vi "I2C Write Byte.vi"(8 "error in (no error)":errorcluster, 10 "Data Byte (0x0)":u8 format="%x", 11 "I2C Task In":T1) -> (0 "error out":errorcluster, 2 "Ack":bool, 3 "I2C Task Out":T1)   [LabVIEW 2017, in "I2C.lvlib"]
doc: "Writes a single byte to an I2C slave device on a single port."
uses:
  <vilib>/robotics/Protocols/I2C/DAQmx/I2C.lvlib
  <vilib>/robotics/Protocols/I2C/DAQmx/Private/I2C Tasks.ctl
  <vilib>/DAQmx/read.llb/DAQmx Read (Digital Bool 1Line 1Point).vi
  <vilib>/DAQmx/miscellaneous.llb/DAQmx Fill In Error Info.vi
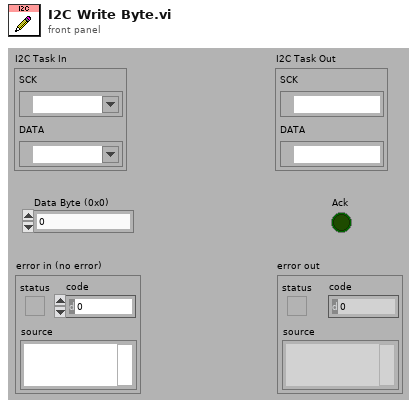
[diagram p1: front panel]
types:
  T1 = typedef "I2C.lvlib/I2C Tasks.ctl" = cluster{"SCK":refnum<k21>, "DATA":refnum<k21>}
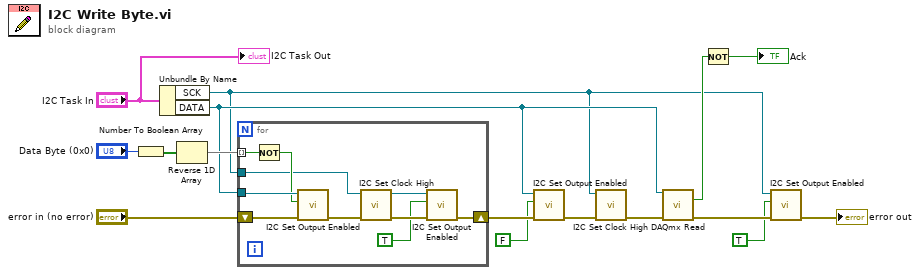
[diagram p0: block diagram]
diagram:
  n1 = Number To Boolean Array(number="Data Byte (0x0)") -> (Boolean array=w16:bool[])
  n2 = Unbundle By Name("I2C Task In") -> ("SCK"=w3:refnum<k21>, "DATA"=w8:refnum<k21>)
  n3 = Reverse 1D Array(array=w16) -> (reversed array=w13:bool[])
  n4 = for {
    tunnel: w13 -> [w26] mode=indexing
    shift-right: [w17] -> w11
    shift-left: "error in (no error)" -> [w25]
    tunnel: w8 -> [w24]
    tunnel: w3 -> [w22]
    n5 = Not(x=w26) -> (.not. x?=w23:bool)
    n6 = call <vilib>:"I2C Set Output Enabled.vi"("error in (no error)"=w25, "Output Enabled (T:Enable)"=w23, "Task In"=w24) -> ("error out"=w21:errorcluster)  [unwired: 7 in, 1 out]
    n7 = call <vilib>:"I2C Set Clock High.vi"("error in (no error)"=w21, "Task In"=w22) -> ("error out"=w19:errorcluster, "Task Out"=w20:refnum<k21>)  [unwired: 8 in]
    n8 = call <vilib>:"I2C Set Output Enabled.vi"("error in (no error)"=w19, "Output Enabled (T:Enable)"=TRUE, "Task In"=w20) -> ("error out"=w17:errorcluster)  [unwired: 7 in, 1 out]
  }
  n9 = call <vilib>:"I2C Set Output Enabled.vi"("error in (no error)"=w11, "Output Enabled (T:Enable)"=FALSE, "Task In"=w8) -> ("error out"=w9:errorcluster)  [unwired: 7 in, 1 out]
  n10 = call <vilib>:"I2C Set Clock High.vi"("error in (no error)"=w9, "Task In"=w3) -> ("error out"=w7:errorcluster)  [unwired: 8 in, 1 out]
  n11 = call-poly <vilib>:"DAQmx Read.vi"("task/channels in"=w8, "error in"=w7) -> ("data"=w6:bool, "error out"=w4:errorcluster)  [unwired: 11 in, 1 out]
  n12 = Not(x=w6) -> (.not. x?=→"Ack":bool)
  n13 = call <vilib>:"I2C Set Output Enabled.vi"("error in (no error)"=w4, "Output Enabled (T:Enable)"=TRUE, "Task In"=w3) -> ("error out"=→"error out":errorcluster)  [unwired: 7 in, 1 out]
  "I2C Task Out" <- "I2C Task In"
